vi "AWS_DataFinder_DisplayResults.vi"(8 "error in":errorcluster, 9 "results elements":T1, 10 "result references":T2[](array[typedef]), 11 "Tbl Refnum":refnum<vi>) -> (0 "error out":errorcluster, 2 "Sensor_Type values":string[](array[string]))   [LabVIEW 2014]
doc: "Fill results table with resulting information."
uses:
  <vilib>/userdefined/DFSearchResult.ctl
  <vilib>/DataFinder/DataTypes/results elements.ctl
  <vilib>/DataFinder/DataTypes/object type.ctl
  <vilib>/DataFinder/DataTypes/property.ctl
  <vilib>/DataFinder/DataTypes/data type.ctl
  <vilib>/DataFinder/Get Property Values (String Property).vi
  <vilib>/DataFinder/NI_DataFinder Toolkit.lvlib
  <vilib>/userdefined/NI_DataFinder Controls.lvlib
panel:
  # "Fill results table with resulting information."
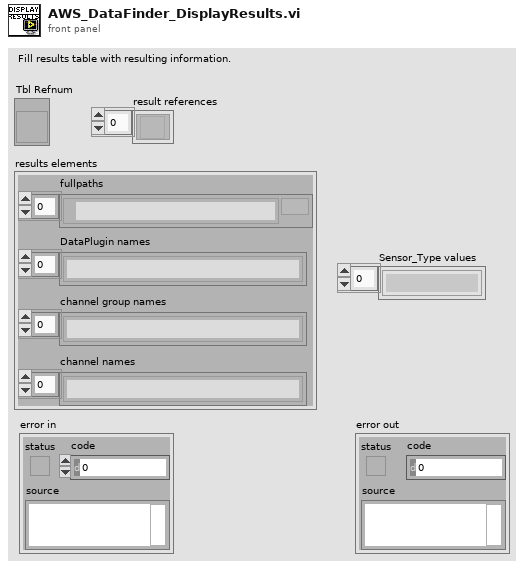
[diagram p1: front panel]
types:
  T1 = typedef "NI_DataFinder Toolkit.lvlib/results elements.ctl" = cluster{"fullpaths":path[], "DataPlugin names":string[], "channel group names":string[], "channel names":string[]}
  T2 = typedef "NI_DataFinder Controls.lvlib/DFSearchResult.ctl" = refnum<k20>
  T3 = typedef "NI_DataFinder Toolkit.lvlib/property.ctl" = cluster{"object type":T4, "property name":string, "data type":T5}
  T4 = typedef "NI_DataFinder Toolkit.lvlib/object type.ctl" = u16
  T5 = typedef "NI_DataFinder Toolkit.lvlib/data type.ctl" = u16
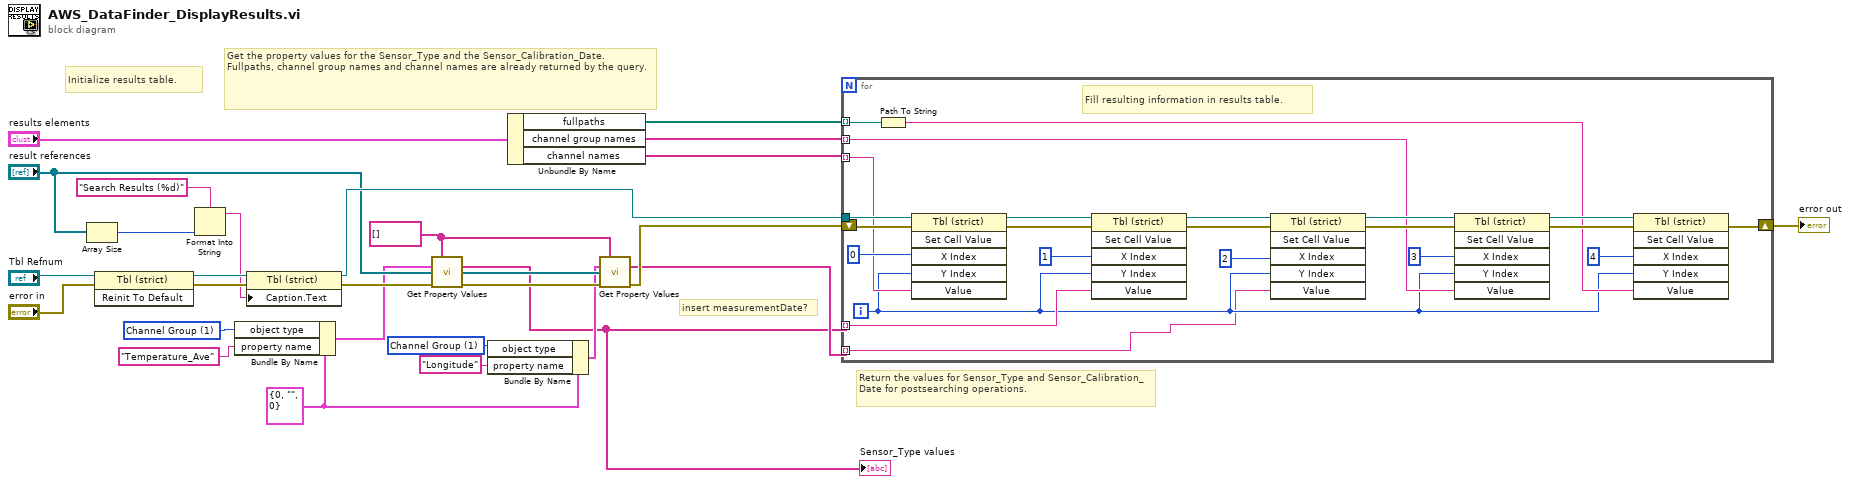
[diagram p0: block diagram]
diagram:
  w8 = T3 {"object type"=0, "property name"="", "data type"=0} ("property")
  w11 = T4 1 items=["File", "Channel Group", "Channel"] ("object type")
  w13 = T4 1 items=["File", "Channel Group", "Channel"] ("object type")
  w2 = string[] [] ("data type")
  # "insert measurementDate?"
  # "Initialize results table."
  # "Return the values for Sensor_Type and Sensor_Calibration_Date for postsearching operations."
  # "Get the property values for the Sensor_Type and the Sensor_Calibration_Date. Fullpaths, channel group names and channel names are already returned by the query."
  n1 = Array Size(array="result references") -> (size(s)=w6:i32)
  n2 = invoke class="Tbl (strict)" method="Reinit To Default"(reference="Tbl Refnum", error in="error in") -> (reference out=w15:refnum<vi>, error out=w16:errorcluster)  [unwired: 1 in, 1 out]
  n3 = Format Into String(format string="Search Results (%d)" ("string"), w6) -> (resulting string=w4:string)  [unwired: 2 in, 1 out]
  n4 = Bundle By Name(cluster=w8, "object type"=w13, "property name"="Temperature_Ave") -> (w12:T3)
  n5 = property class="Tbl (strict)"(reference=w15, error in=w16, "Caption.Text"=w4) -> (reference out=w23:refnum<vi>, error out=w22:errorcluster)
  n6 = call-poly <vilib>:"Get Property Values.vi"("data type"=w2, "property"=w12, "result references"="result references", "error in (no error)"=w22) -> ("property values"=w7:string[], "result references out"=w20:T2[], "error out"=w19:errorcluster)  [unwired: 9 out]
  "Sensor_Type values" <- w7
  n7 = Bundle By Name(cluster=w8, "object type"=w11, "property name"="Longitude") -> (w10:T3)
  n8 = Unbundle By Name("results elements") -> ("fullpaths"=w26:path[], "channel group names"=w1:string[], "channel names"=w14:string[])
  n9 = call-poly <vilib>:"Get Property Values.vi"("data type"=w2, "property"=w10, "result references"=w20, "error in (no error)"=w19) -> ("property values"=w17:string[], "error out"=w18:errorcluster)  [unwired: 10 out]
  n10 = for {
    shift-right: [w40] -> w28
    shift-left: w18 -> [w50]
    tunnel: w1 -> [w32] mode=indexing
    tunnel: w26 -> [w34] mode=indexing
    tunnel: w23 -> [w43]
    tunnel: w7 -> [w33] mode=indexing
    tunnel: w17 -> [w29] mode=indexing
    tunnel: w14 -> [w35] mode=indexing
    i -> [w30]
    # "Fill resulting information in results table."
    n11 = Path To String(path=w34) -> (string=w31:string)
    n12 = invoke on="Invoke Node" class="Tbl (strict)" method="Set Cell Value"(reference=w43, error in=w50, "X Index"=u32 0, "Y Index"=w30, "Value"=w35) -> (reference out=w48:refnum<vi>, error out=w49:errorcluster)  [unwired: 1 in, 4 out]
    n13 = invoke on="Invoke Node" class="Tbl (strict)" method="Set Cell Value"(reference=w48, error in=w49, "X Index"=u32 1, "Y Index"=w30, "Value"=w33) -> (reference out=w44:refnum<vi>, error out=w45:errorcluster)  [unwired: 1 in, 4 out]
    n14 = invoke on="Invoke Node" class="Tbl (strict)" method="Set Cell Value"(reference=w44, error in=w45, "X Index"=u32 2, "Y Index"=w30, "Value"=w29) -> (reference out=w37:refnum<vi>, error out=w36:errorcluster)  [unwired: 1 in, 4 out]
    n15 = invoke on="Invoke Node" class="Tbl (strict)" method="Set Cell Value"(reference=w37, error in=w36, "X Index"=u32 3, "Y Index"=w30, "Value"=w32) -> (reference out=w38:refnum<vi>, error out=w39:errorcluster)  [unwired: 1 in, 4 out]
    n16 = invoke on="Invoke Node" class="Tbl (strict)" method="Set Cell Value"(reference=w38, error in=w39, "X Index"=u32 4, "Y Index"=w30, "Value"=w31) -> (error out=w40:errorcluster)  [unwired: 1 in, 5 out]
  }
  "error out" <- w28
